vi "IMD Test Settings Get Configuration Data.vi"(8 "error in":errorcluster, 10 "Configuration Name":string, 11 "IMD Test Settings in":refnum<class "IMD Test Settings.lvclass">) -> (0 "error IO":errorcluster, 2 "IMD Settings Cluster":T1, 3 "IMD Test Settings out":refnum<class "IMD Test Settings.lvclass">)   [LabVIEW 2016, in "IMD Test Settings.lvlib" / "IMD Test Settings.lvclass"]
uses:
  IMD Test Settings.lvclass
  C:/Projects/STS/Common/Sequence Automation/Plugins/Test Settings/ITestSettings.lvlibp/ITestSettings.lvclass
  Controls/IMD Settings Cluster.ctl
  Plugins/Test Settings/ITestSettings.lvlibp/Protected Methods/Read Configuration Dictionary.vi
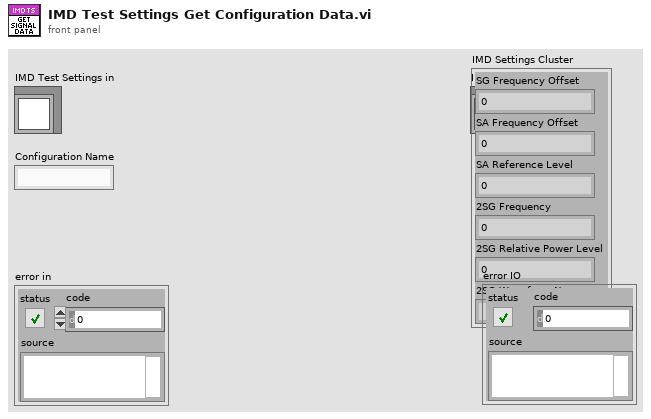
[diagram p1: front panel]
types:
  T1 = typedef "IMD Test Settings.lvlib/IMD Test Settings.lvclass/IMD Settings Cluster.ctl" = cluster{"SG Frequency Offset":dbl, "SA Frequency Offset":dbl, "SA Reference Level":dbl, "2SG Frequency":dbl, "2SG Relative Power Level":dbl, "2SG Waveform Name":string}
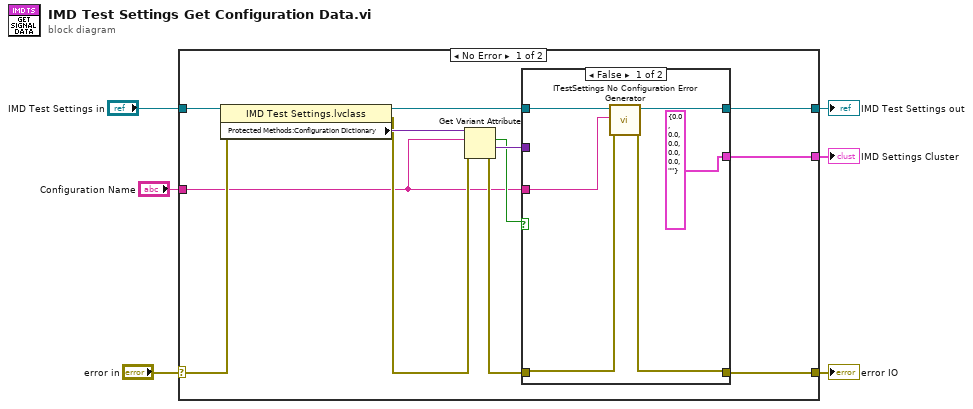
[diagram p0: block diagram]
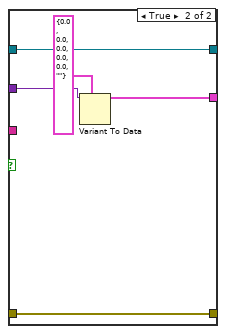
[diagram p2: hidden frame]
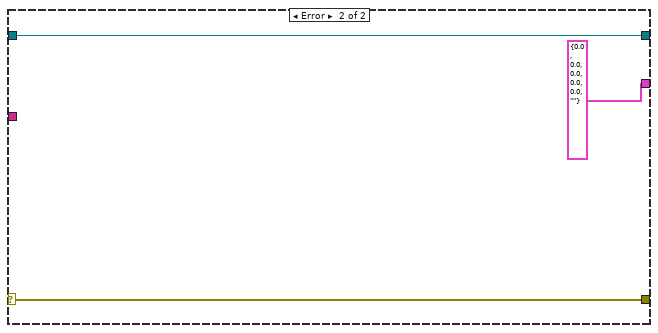
[diagram p3: hidden frame]
diagram:
  n1 = case shown="No Error" "error in" {
    selector: "error in" -> [w18 w32]
    tunnel: [w8 w32] -> w1
    tunnel: [w9 w31] -> w3
    tunnel: "IMD Test Settings in" -> [w17 w31]
    tunnel: "Configuration Name" -> [w7 _]
    tunnel: [w13 T1 {"SG Frequency Offset"=0.0, "SA Frequency Offset"=0.0, "SA Reference Level"=0.0, "2SG Frequency"=0.0, "2SG Relative Power Level"=0.0, "2SG Waveform Name"=""} ("IMD Settings Cluster")] -> w2
    frame No Error {
      n2 = property class="IMD Test Settings.lvclass"(reference=w17, error in=w18) -> (reference out=w10:refnum<class "IMD Test Settings.lvclass">, error out=w15:errorcluster, "Protected Methods:Configuration Dictionary"=w16:variant)
      n3 = Get Variant Attribute(Variant=w16, name=w7, error in=w15) -> (found=w12:bool, value=w14:variant, error out=w11:errorcluster)  [unwired: 1 in, 1 out]
      n4 = case shown="False" w12 {
        tunnel: w14 -> [_ w29]
        tunnel: [T1 {"SG Frequency Offset"=0.0, "SA Frequency Offset"=0.0, "SA Reference Level"=0.0, "2SG Frequency"=0.0, "2SG Relative Power Level"=0.0, "2SG Waveform Name"=""} ("IMD Settings Cluster") w28] -> w13
        tunnel: w11 -> [w22 w26]
        tunnel: w10 -> [w24 w27]
        tunnel: [w23 w27] -> w9
        tunnel: [w21 w26] -> w8
        tunnel: w7 -> [w20 _]
        frame False {
          n5 = call-dynamic "ITestSettings No Configuration Error Generator.vi"("error in (no error)"=w22, "Configuration In"=w20, "ITestSettings in"=w24) -> ("error out"=w21:errorcluster, "ITestSettings out"=w23:refnum<class "IMD Test Settings.lvclass">)  [unwired: 7 in]
        }
        frame True {
          n6 = Variant To Data(type=T1 {"SG Frequency Offset"=0.0, "SA Frequency Offset"=0.0, "SA Reference Level"=0.0, "2SG Frequency"=0.0, "2SG Relative Power Level"=0.0, "2SG Waveform Name"=""} ("IMD Settings Cluster"), Variant=w29) -> (data=w28:T1)  [unwired: 1 in, 1 out]
        }
      }
    }
    frame Error {
    }
  }
  "IMD Test Settings out" <- w3
  "IMD Settings Cluster" <- w2
  "error IO" <- w1
